vi "Get control from cluster.vi"(8 "Mapping array":i8[](array[numeric]), 9 "Combo Box":string(combo), 10 "Array of booleans":string[](array[string]), 11 "Controls[]":refnum<vi>[](array[refnum])) -> (3 "control ref":refnum<vi>)   [LabVIEW 2015]
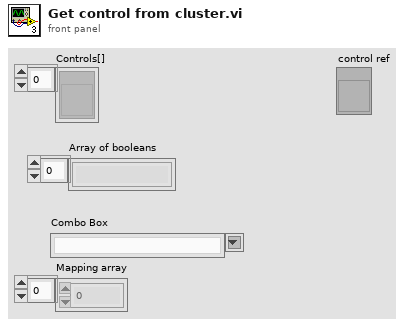
[diagram p1: front panel]
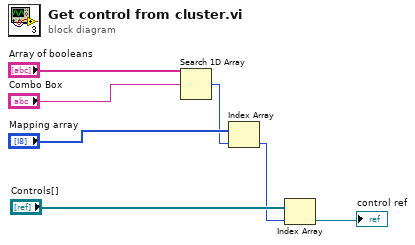
[diagram p0: block diagram]
diagram:
  n1 = Search 1D Array(1D array="Array of booleans", element="Combo Box") -> (index of element=w4:i32)  [unwired: 1 in]
  n2 = Index Array(array="Mapping array", index=w4) -> (element=w2:i8)
  n3 = Index Array(array="Controls[]", index=w2) -> (element=→"control ref":refnum<vi>)
